vi "Write TestCases.vi"(5 "TestCases":refnum<class "TestCase.lvclass">[](array[class]), 9 "TestSuite in":refnum<class "TestSuite.lvclass">) -> (3 "TestSuite out":refnum<class "TestSuite.lvclass">)   [LabVIEW 2014, in "TestSuite.lvclass"]
uses:
  TestSuite.lvclass
  TestCase/TestCase.lvclass
  TestSuite.lvclass/TestSuite.ctl
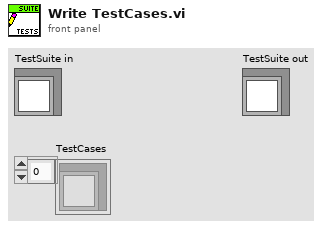
[diagram p1: front panel]
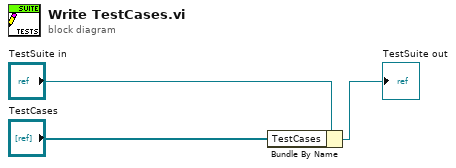
[diagram p0: block diagram]
diagram:
  n1 = Bundle By Name(cluster="TestSuite in", "TestCases"="TestCases") -> (→"TestSuite out":refnum<class "TestSuite.lvclass">)
